vi "write processed data to network stream.vi"(9 "Data":T1={"Parameters"={"FPGA Ref"=refnum, "data stream"={"data writer name"="error writer", "NS write buffer size"=16, "NS Buffer length"=0}, "FIFO Depth"=0, "Channel controls"={"FIFO channel count"=0, "active indices"=[], "active channels"=0, "channelScaling"=[], "scanivalveCount"=0, "channels"=[]}, "safetyChannels"={"oilP"=0, "airP"=0, "water"=0, "channelLimits"=[]}, "speedChannel"=0, "maxSpeedLimit"=0.0, "Torque"={"fixedOffset"=0.0, "filter"=FALSE, "fallingEdge"=FALSE, "swapEncoders"=FALSE}}, "Variables"={"Intermediary buffer"=[], "buffer position"=0, "write loop counter"=0, "NS write trigger"=0, "NS Connection status"=FALSE, "waiting for NS"=FALSE, "labAmbient"={"pressure"=0.0, "temperature"=0.0}, "scanivalvePorts"=[], "scanivalvePressures"=[], "data stream"="", "activeChannelLimitIndex"=[], "runningSpeedLimit"=0.0, "speedChannelIndex"=0, "Interlocks"={"gearboxOil"=FALSE, "bearingOil"=FALSE, "gearboxAir"=FALSE}, "interlockChannels"={"gearboxOil"=0, "bearingOil"=0, "air"=0}, "limitStates"=[]}}, 11 "RT Queues":T8) -> (1 "Data out":T1={"Parameters"={"FPGA Ref"=refnum, "data stream"={"data writer name"="error writer", "NS write buffer size"=16, "NS Buffer length"=0}, "FIFO Depth"=0, "Channel controls"={"FIFO channel count"=0, "active indices"=[], "active channels"=0, "channelScaling"=[], "scanivalveCount"=0, "channels"=[]}, "safetyChannels"={"oilP"=0, "airP"=0, "water"=0, "channelLimits"=[]}, "speedChannel"=0, "maxSpeedLimit"=0.0, "Torque"={"fixedOffset"=0.0, "filter"=FALSE, "fallingEdge"=FALSE, "swapEncoders"=FALSE}}, "Variables"={"Intermediary buffer"=[], "buffer position"=0, "write loop counter"=0, "NS write trigger"=0, "NS Connection status"=FALSE, "waiting for NS"=FALSE, "labAmbient"={"pressure"=0.0, "temperature"=0.0}, "scanivalvePorts"=[], "scanivalvePressures"=[], "data stream"="", "activeChannelLimitIndex"=[], "runningSpeedLimit"=0.0, "speedChannelIndex"=0, "Interlocks"={"gearboxOil"=FALSE, "bearingOil"=FALSE, "gearboxAir"=FALSE}, "interlockChannels"={"gearboxOil"=0, "bearingOil"=0, "air"=0}, "limitStates"=[]}})   [LabVIEW 2018]
uses:
  Type Defs/Queues cluster.ctl
  ICL-LabVIEW_General/Message Scheduler/message scheduler.lvclass
  Type Defs/Data processing loop data.ctl
  Type Defs/FPGA reference.ctl
  PC/type defs/channelControl.ctl
  Type Defs/channelScalingTypes.ctl
  Type Defs/scalingMethods.ctl
  ICL-LabVIEW_General/data channels/parent class/Data Channel.lvclass
  PC/type defs/channelLimitControl.ctl
  PC/type defs/limitActions.ctl
  <vilib>/Utility/error.llb/Error Cluster From Error Code.vi
  Queue VIs/En-queue RT data element.vi
  <vilib>/ErrorRing/Error Ring.xnode
  <resource>/objmgr/ni.dex.rc
panel:
  out "time":dbl
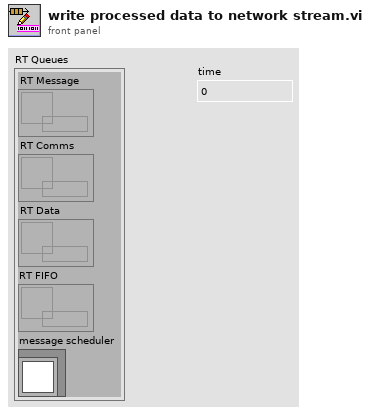
[diagram p1: front panel]
types:
  T1 = typedef "Data processing loop data.ctl" = cluster{"Parameters":cluster{"FPGA Ref":T2, "data stream":cluster{"data writer name":string, "NS write buffer size":i32, "NS Buffer length":u32}, "FIFO Depth":u32, "Channel controls":cluster{"FIFO channel count":i32, "active indices":i16[], "active channels":i32, "channelScaling":T3[], "scanivalveCount":i32, "channels":refnum<class "Data Channel.lvclass">[]}, "safetyChannels":cluster{"oilP":u16, "airP":u16, "water":u16, "channelLimits":T6[]}, "speedChannel":i32, "maxSpeedLimit":dbl, "Torque":cluster{"fixedOffset":dbl, "filter":bool, "fallingEdge":bool, "swapEncoders":bool}}, "Variables":cluster{"Intermediary buffer":dbl[][], "buffer position":u32, "write loop counter":u16, "NS write trigger":u32, "NS Connection status":bool, "waiting for NS":bool, "labAmbient":cluster{"pressure":dbl, "temperature":dbl}, "scanivalvePorts":u16[], "scanivalvePressures":dbl[], "data stream":refnum<k21>, "activeChannelLimitIndex":u16[], "runningSpeedLimit":dbl, "speedChannelIndex":i32, "Interlocks":cluster{"gearboxOil":bool, "bearingOil":bool, "gearboxAir":bool}, "interlockChannels":cluster{"gearboxOil":i32, "bearingOil":i32, "air":i32}, "limitStates":cluster{"warn":bool, "alarm":bool}[]}}
  T2 = typedef "FPGA reference.ctl" = refnum<k20>
  T3 = typedef "channelControl.ctl" = cluster{"index":u16, "active":bool, "channelType":T4, "module":u16, "terminal":u16, "channelName":string, "scalingMethod":T5, "scalingParameters":dbl[], "scaledUnits":string, "tempOffset":dbl}
  T4 = typedef "channelScalingTypes.ctl" = enum16{"calculation", "measurement", "scanivalve", "output", "digital"}
  T5 = typedef "scalingMethods.ctl" = enum16{"none", "linear", "thermocouple", "polynomial", "encoder", "RTD"}
  T6 = typedef "channelLimitControl.ctl" = cluster{"channelID":u16, "Enabled":bool, "warnValue":dbl, "limitValue":dbl, "Invert":bool, "limitAction":T7}
  T7 = typedef "limitActions.ctl" = enum16{"stop", "shutdown", "ignore"}
  T8 = typedef "Queues cluster.ctl" = cluster{"RT Message":refnum<queue>, "RT Comms":refnum<queue>, "RT Data":refnum<queue>, "RT FIFO":refnum<queue>, "message scheduler":refnum<class "message scheduler.lvclass">}
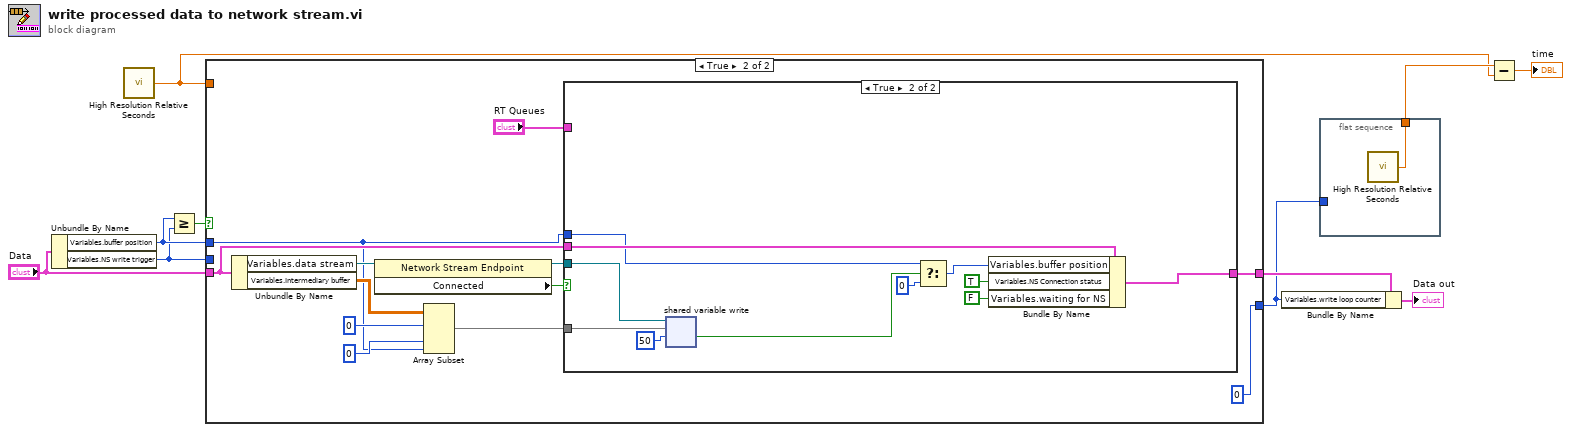
[diagram p0: block diagram]
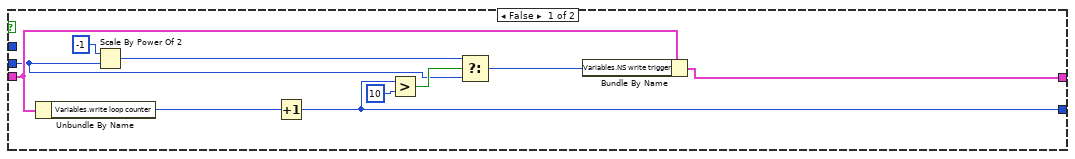
[diagram p2: hidden frame]
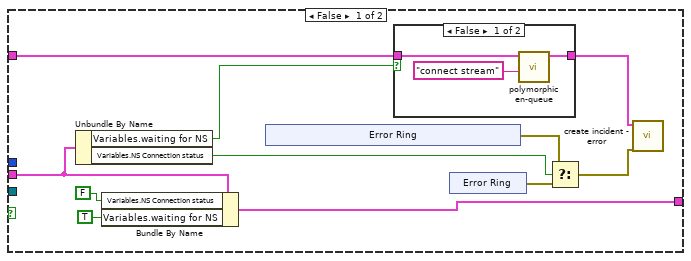
[diagram p3: hidden frame]
diagram:
  n1 = Unbundle By Name("Data") -> ("Variables.buffer position"=w8:u32, "Variables.NS write trigger"=w5:u32)
  n2 = call <vilib>:"High Resolution Relative Seconds.vi"() -> ("relative seconds"=w2:dbl)
  n3 = Greater Or Equal?(x=w8, y=w5) -> (x >= y?=w7:bool)
  n4 = case shown="True" w7 {
    tunnel: [w17 w25] -> w10
    tunnel: "Data" -> [w18 w23]
    tunnel: w8 -> [_ w22]
    tunnel: [w11 u16 0 ("Variables.write loop counter")] -> w4
    tunnel: w5 -> [w13 _]
    tunnel: w2 -> [_ _]
    frame False {
      n5 = Unbundle By Name(w18) -> ("Variables.write loop counter"=w20:u16)
      n6 = Scale By Power Of 2(n=i16 -1, x=w13) -> (x*2^n=w14:u32)
      n7 = Increment(x=w20) -> (x+1=w11:u16)
      n8 = Greater?(x=w11, y=u16 10) -> (0:w15:bool)
      n9 = Select(t=w14, s=w15, f=w13) -> (s? t:f=w12:u32)
      n10 = Bundle By Name(cluster=w18, "Variables.NS write trigger"=w12) -> (w17:T1)
    }
    frame True {
      n11 = Unbundle By Name(w23) -> ("Variables.data stream"=w32:refnum<k21>, "Variables.Intermediary buffer"=w29:dbl[][])
      n12 = property class="Network Stream Endpoint"(reference=w32) -> (reference out=w30:refnum<k21>, "Connected"=w31:bool)  [unwired: 1 in, 1 out]
      n13 = Array Subset(array=w29, index (row)=0 ("index"), index (col)=0 ("index"), length (col)=w22) -> (w26:dbl[][])  [unwired: 1 in]
      n14 = case shown="True" w31 {
        tunnel: w30 -> [_ w64]
        tunnel: w26 -> [_ w62]
        tunnel: w23 -> [w39 w61]
        tunnel: [w41 w60] -> w25
        tunnel: "RT Queues" -> [w43 _]
        tunnel: w22 -> [_ w58]
        frame False {
          n15 = Unbundle By Name(w39) -> ("Variables.waiting for NS"=w34:bool, "Variables.NS Connection status"=w38:bool)
          n16 = Bundle By Name(cluster=w39, "Variables.NS Connection status"=FALSE, "Variables.waiting for NS"=TRUE) -> (w41:T1)
          n17 = xnode "Error Ring"() -> ("error out"=w37:errorcluster)
          n18 = case shown="False" w34 {
            tunnel: w43 -> [w46 w47]
            tunnel: [w44 w47] -> w42
            frame False {
              n19 = call-poly "polymorphic en-queue.vi"("Message"="connect stream", "RT Queues"=w46) -> ("RT Queues out"=w44:T8)  [unwired: 7 in, 2 out]
            }
            frame True {
            }
          }
          n20 = xnode "Error Ring"() -> ("error out"=w35:errorcluster)
          n21 = Select(t=w37, s=w38, f=w35) -> (s? t:f=w36:errorcluster)
          n22 = call "create incident - error.vi"("error"=w36, "RT Queues"=w42) -> ()  [unwired: 9 in, 1 out]
        }
        frame True {
          n23 = shared-variable-write(w64, w62, 50 ("timeout ms (-1)")) -> (w59:bool)  [unwired: 1 in, 2 out]
          n24 = Select(t=w58, s=w59, f=u32 0 ("Variables.buffer position")) -> (s? t:f=w56:u32)
          n25 = Bundle By Name(cluster=w61, "Variables.buffer position"=w56, "Variables.NS Connection status"=TRUE, "Variables.waiting for NS"=FALSE) -> (w60:T1)
        }
      }
    }
  }
  n26 = Bundle By Name(cluster=w10, "Variables.write loop counter"=w4) -> (→"Data out":T1)
  n27 = flat-sequence {
    tunnel: w4 -> [_]
    tunnel: [w65] -> w3
    frame #0 {
      n28 = call <vilib>:"High Resolution Relative Seconds.vi"() -> ("relative seconds"=w65:dbl)
    }
  }
  n29 = Subtract(x=w3, y=w2) -> (x-y=→"time":dbl)
